vi "manual.vi"(0 "DI7":bool, 5 "DI8":bool, 7 "DI9":bool, 9 "DI10":bool, 11 "DI11":bool, 12 "DI12":bool, 13 "DI13":bool) -> (4 "DO2":bool, 6 "DO3":bool, 8 "DO4":bool, 10 "DO5":bool, 15 "DO6":bool)   [LabVIEW 2019]
panel:
  out "DI13":bool
  out "DI12":bool
  out "DI11":bool
  out "DI10":bool
  out "DI9":bool
  out "DI8":bool
  out "DI7":bool
  in  "DO6":bool
  in  "DO5":bool
  in  "DO4":bool
  in  "DO3":bool
  in  "DO2":bool
  # "CONTORL MANUAL"
  # "ENTRADAS"
  # "SALIDAS"
  # "BYPASS"
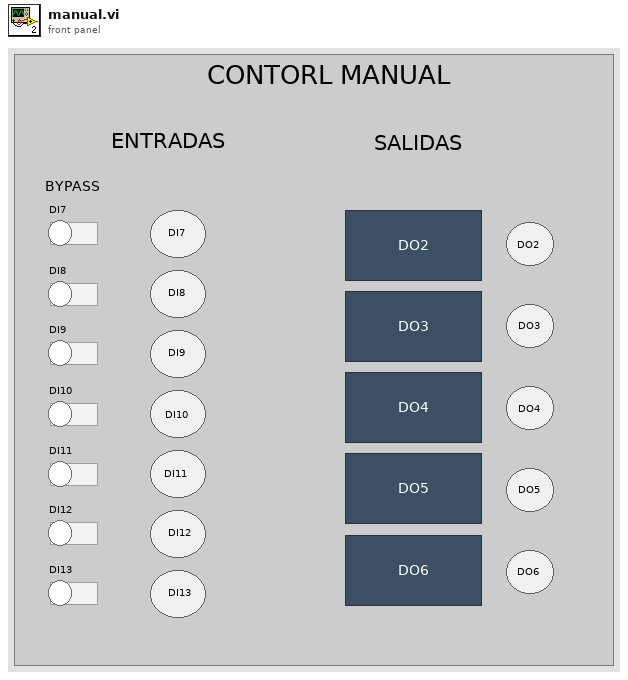
[diagram p1: front panel]
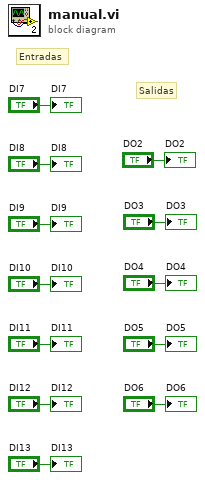
[diagram p0: block diagram]
diagram:
  # "Salidas"
  # "Entradas"
  "DI7" <- "DI7"
  "DO2" <- "DO2"
  "DO3" <- "DO3"
  "DO4" <- "DO4"
  "DO5" <- "DO5"
  "DO6" <- "DO6"
  "DI8" <- "DI8"
  "DI9" <- "DI9"
  "DI10" <- "DI10"
  "DI11" <- "DI11"
  "DI12" <- "DI12"
  "DI13" <- "DI13"
